vi "Measure_Gain.vi"(1 "Frequency (MHz)":dbl) -> (0 "Gain (dB)":dbl)   [LabVIEW 2026]
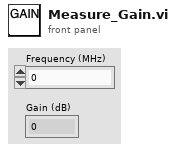
[diagram p1: front panel]
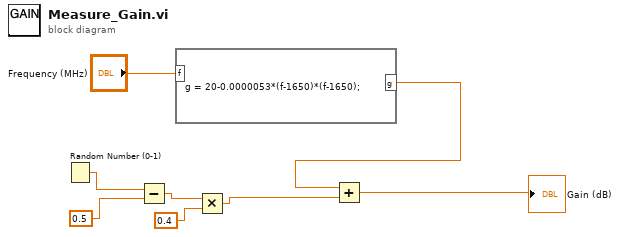
[diagram p0: block diagram]
diagram:
  n1 = Random Number (0-1)() -> (number: 0 to 1=w6:dbl)
  n2 = Subtract(x=w6, y=0.5) -> (x-y=w5:dbl)
  n3 = formula code="g = 20-0.0000053*(f-1650)*(f-1650);"("f"="Frequency (MHz)") -> ("g"=w3:dbl)
  n4 = Multiply(x=w5, y=0.4) -> (x*y=w2:dbl)
  n5 = Add(x=w3, y=w2) -> (x+y=→"Gain (dB)":dbl)
